vi "fileRead.vi"() -> ()   [LabVIEW 2023]
panel:
  out "Right data read string output":string
  in  "stop 2":bool
  in  "Initialize data read for right side":bool
  in  "Initialize data read for left side":bool
  out "Left data read string output":string
  in  "stop":bool
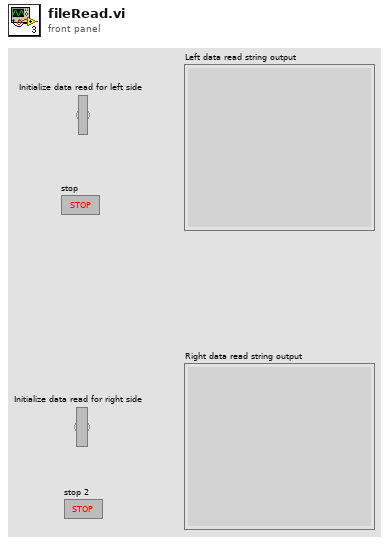
[diagram p1: front panel]
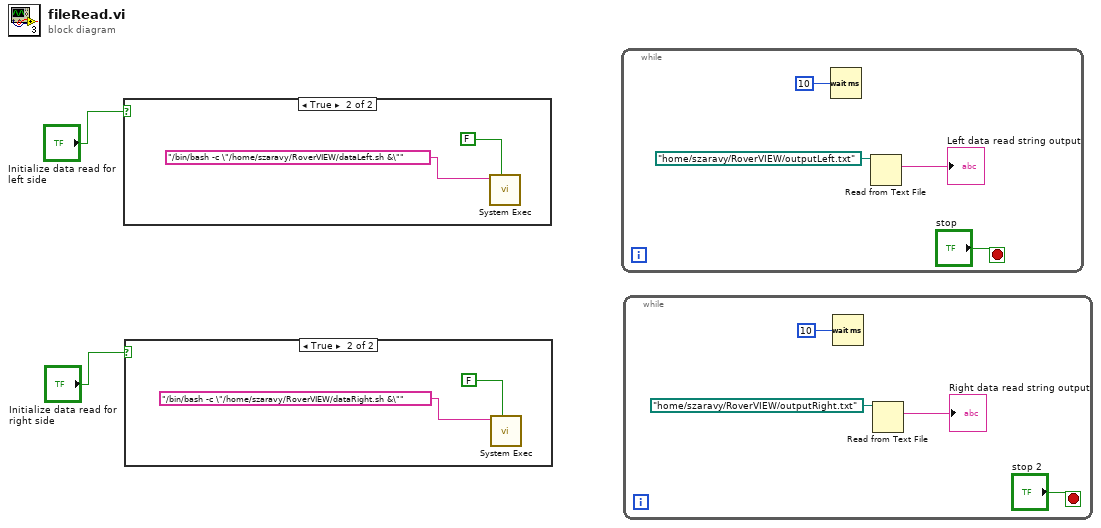
[diagram p0: block diagram]
diagram:
  n1 = case shown="True" "Initialize data read for left side" {
    frame False {
    }
    frame True {
      n2 = call <vilib>:"System Exec.vi"("wait until completion? (T)"=FALSE, "command line"="/bin/bash -c \"/home/szaravy/RoverVIEW/dataLeft.sh &\"") -> ()  [unwired: 6 in, 4 out]
    }
  }
  n3 = case shown="True" "Initialize data read for right side" {
    frame False {
    }
    frame True {
      n4 = call <vilib>:"System Exec.vi"("wait until completion? (T)"=FALSE, "command line"="/bin/bash -c \"/home/szaravy/RoverVIEW/dataRight.sh &\"") -> ()  [unwired: 6 in, 4 out]
    }
  }
  n5 = while {
    stop <- "stop" stop-if-true
    n6 = Wait (ms)(milliseconds to wait=u32 10) -> ()  [unwired: 1 out]
    n7 = Read from Text File(file (use dialog)=path "/home/szaravy/RoverVIEW/outputLeft.txt") -> (text=→"Left data read string output":string)  [unwired: 3 in, 3 out]
  }
  n8 = while {
    stop <- "stop 2" stop-if-true
    n9 = Wait (ms)(milliseconds to wait=u32 10) -> ()  [unwired: 1 out]
    n10 = Read from Text File(file (use dialog)=path "/home/szaravy/RoverVIEW/outputRight.txt") -> (text=→"Right data read string output":string)  [unwired: 3 in, 3 out]
  }
